vi "UIRefs Button Switch.vi"(8 "error in (no error)":errorcluster, 11 "Valve in":refnum<class "Valve.lvclass">) -> (0 "error out":errorcluster, 3 "Valve out":refnum<class "Valve.lvclass">)   [LabVIEW 2021, in "Valve.lvlib" / "Valve.lvclass"]
uses:
  Valve.lvclass
  Valve.lvclass/Valve.ctl
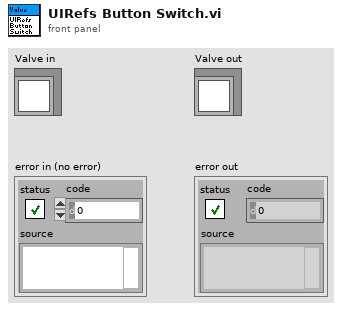
[diagram p1: front panel]
types:
  T1 = enum8{"Enabled", "Disabled", "Disabled and Grayed Out"}
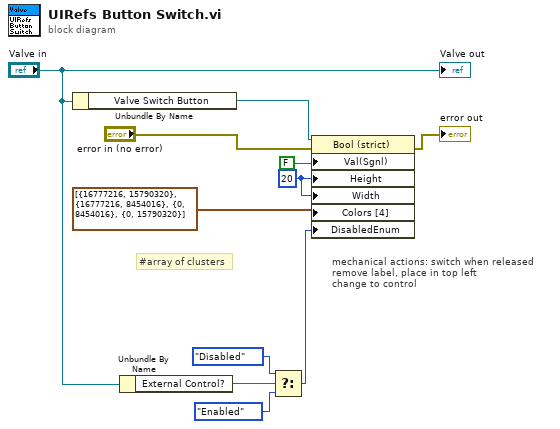
[diagram p0: block diagram]
diagram:
  w10 = u32 20 ("Button Size:Height")
  # "#array of clusters"
  # "mechanical actions: switch when released\nremove label, place in top left\nchange to control"
  n1 = Unbundle By Name("Valve in") -> ("Valve Switch Button"=w6:refnum<vi>)
  n2 = Unbundle By Name("Valve in") -> ("External Control?"=w4:bool)
  n3 = Select(t=T1."Disabled" ("Disabled"), s=w4, f=T1."Enabled" ("Disabled")) -> (s? t:f=w1:T1)
  n4 = property class="Bool (strict)"(reference=w6, error in="error in (no error)", "Val(Sgnl)"=FALSE ("Value (Signaling)"), "Height"=w10, "Width"=w10, "Colors [4]"=cluster{u32, u32}[] [{16777216, 15790320}, {16777216, 8454016}, {0, 8454016}, {0, 15790320}], "DisabledEnum"=w1) -> (error out=→"error out":errorcluster)  [unwired: 1 out]
  "Valve out" <- "Valve in"
